vi "BuildMask_Blue.vi"(2 "threshold":cluster{u8, u8}(slide)={23, 255} scale=0.0..255.0, 3 "Image":T1 {"Dialogs" format="%.0b"}) -> (1 "Image":T1 {"Dialogs" format="%.0b"})   [LabVIEW 2010]
doc: "This vi will return a mask. The area inside the defined ROI is filled with 255 and the rest of the image is set to 0."
uses:
  <userlib>/ImageProcessing/QTLIB_2595_LV86/QT_Image.ctl
panel:
  # "This vi will return a mask.  The area inside the defined ROI is filled with 255 and the rest of the image is set to 0."
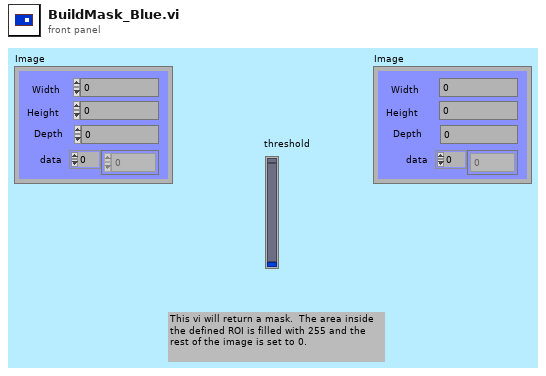
[diagram p1: front panel]
types:
  T1 = typedef "QT_Image.ctl" = cluster{"Width":i32, "Height":i32, "Depth":i32, "data":u8[], "Compressed data":u8[], "Color table":u32[], "Duration":i32, "Options":i32, "Timestamp":i32, "ID":i32, "Reserved":i32, "Dialogs":u32}
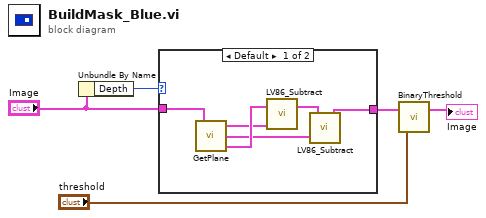
[diagram p0: block diagram]
diagram:
  n1 = Unbundle By Name("Image") -> ("Depth"=w4:i32)
  n2 = case shown="Default" w4 {
    tunnel: [w9 w12] -> w2
    tunnel: "Image" -> [w11 w12]
    frame Default {
      n3 = call <userlib>:"GetPlane.vi"("Image In"=w11) -> ("Blue Plane Out"=w8:T1, "Green Plane Out"=w6:T1, "Red Plane Out"=w7:T1)
      n4 = call <userlib>:"LV86_Subtract.vi"("Image 2"=w7, "Image"=w8) -> ("Image Out"=w10:T1)  [unwired: 1 in]
      n5 = call <userlib>:"LV86_Subtract.vi"("Image 2"=w6, "Image"=w10) -> ("Image Out"=w9:T1)  [unwired: 1 in]
    }
    frame 1, 8 {
    }
  }
  n6 = call <userlib>:"BinaryThreshold.vi"("threshold"="threshold", "Image In"=w2) -> ("Image Out"=→"Image":T1)  [unwired: 1 in]
